vi "Check Position.vi"(8 "error in (no error)":errorcluster, 9 "Start (True)":bool=TRUE, 10 "Count (10000)":i32=10000, 11 "Point In (0)":i32) -> (0 "error out":errorcluster, 3 "Point Out":i32=1)   [LabVIEW 2011, in "Tektronix 7000 Series.lvlib"]
doc: "This VI is used to check the input point or end point is available."
uses:
  Tektronix 7000 Series.lvlib
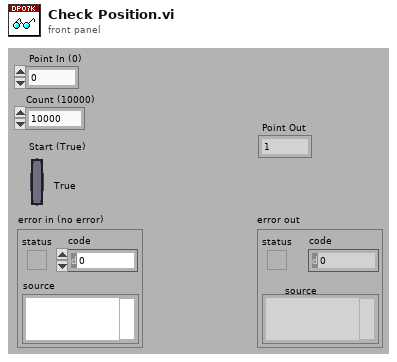
[diagram p1: front panel]
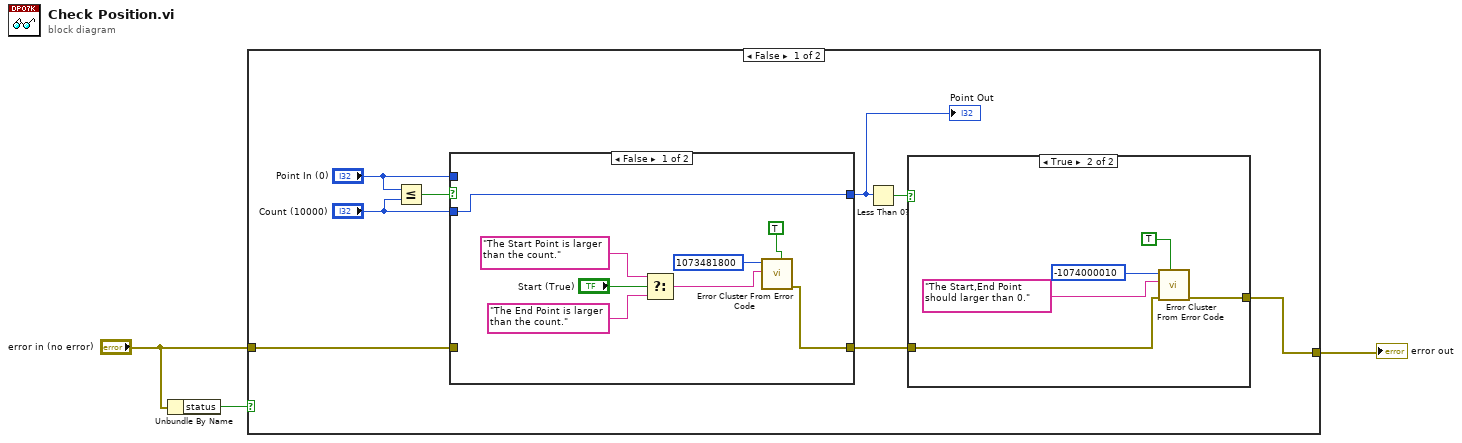
[diagram p0: block diagram]
diagram:
  n1 = Unbundle By Name("error in (no error)") -> ("status"=w3:bool)
  n2 = case shown="False" w3 {
    tunnel: [w5 w28] -> w2
    tunnel: "error in (no error)" -> [w7 w28]
    frame False {
      n3 = Less Or Equal?(x="Point In (0)", y="Count (10000)") -> (x <= y?=w8:bool)
      n4 = case shown="False" w8 {
        tunnel: [w25 w27] -> w4
        tunnel: "Point In (0)" -> [_ w27]
        tunnel: "Count (10000)" -> [w25 _]
        tunnel: w7 -> [_ w26]
        tunnel: [w20 w26] -> w6
        frame False {
          n5 = Select(t="The Start Point is larger than the count." ("Source"), s="Start (True)", f="The End Point is larger than the count." ("Source")) -> (s? t:f=w19:string)
          n6 = call <vilib>:"Error Cluster From Error Code.vi"("is warning? (False)"=TRUE ("show call chain? (False)"), "error message (\"\")"=w19, "error code (0)"=1073481800 ("Code")) -> ("error out"=w20:errorcluster)  [unwired: 6 in]
        }
        frame True {
        }
      }
      "Point Out" <- w4
      n7 = Less Than 0?(x=w4) -> (x < 0?=w11:bool)
      n8 = case shown="True" w11 {
        tunnel: w6 -> [w12 w15]
        tunnel: [w12 w14] -> w5
        frame False {
        }
        frame True {
          n9 = call <vilib>:"Error Cluster From Error Code.vi"("show call chain? (False)"=TRUE, "error in (no error)"=w15, "error message (\"\")"="The Start,End Point should larger than 0." ("Source"), "error code (0)"=-1074000010 ("Code")) -> ("error out"=w14:errorcluster)  [unwired: 5 in]
        }
      }
    }
    frame True {
    }
  }
  "error out" <- w2
